vi "Configure_Voltage_Range.vi"(6 "Measurement Type":T2(ring), 8 "error in (no error)":errorcluster, 9 "Resolution in Digits":T1(ring), 10 "Range":dbl=1.2, 11 "NI-DCPower in":refnum<class "niDCPower.lvclass">) -> (0 "error out":errorcluster, 3 "NI-DCpower out":refnum<class "niDCPower.lvclass">)   [LabVIEW 2021, in "niDCPower.lvclass"]
uses:
  niDCPower.lvclass
  <instrlib>/niDCPower/nidcpower.llb/niDCPower Source Mode.ctl
  niDCPower.lvclass/niDCPower.ctl
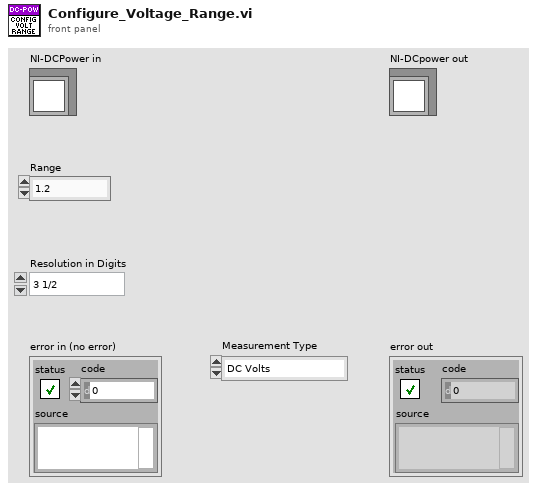
[diagram p1: front panel]
types:
  T1 = enum32{"3 1/2", "4 1/2", "5 1/2", "6 1/2", "7 1/2"}
  T2 = enum32{"DC Volts", "AC Volts", "DC Current", "AC Current", "2-wire Resistance", "4-wire Resistance", "Diode", "Frequency", "Period", "AC Volts DC Coupled", "Capacitance", "Inductance", "Temperature"}
  T3 = typedef "niDCPower Source Mode.ctl" = i32
  T4 = typedef "niDCPower Output Function.ctl" = i32
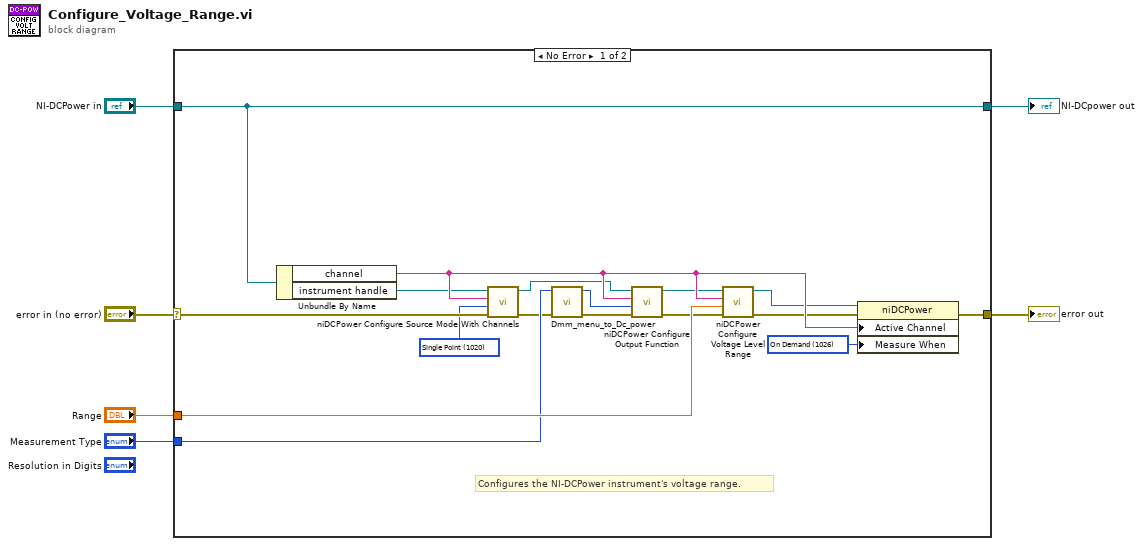
[diagram p0: block diagram]
diagram:
  n1 = case shown="No Error" "error in (no error)" {
    selector: "error in (no error)" -> [w23 w24]
    tunnel: [w22 w24] -> w5
    tunnel: "NI-DCPower in" -> [w19 w25]
    tunnel: [w19 w25] -> w3
    tunnel: "Range" -> [w21 _]
    tunnel: "Measurement Type" -> [w20 _]
    frame No Error {
      w12 = 1026 items=["Automatically after Source Complete"=1025, "On Demand"=1026, "On Measure Trigger"=1027] ("Measurement:Advanced:Measure When")
      w13 = T3 1020 items=["Single Point"=1020, "Sequence"=1021] ("source mode")
      # "Configures the NI-DCPower instrument's voltage range."
      n2 = Unbundle By Name(w19) -> ("channel"=w18:string, "instrument handle"=w17:refnum<k15>)
      n3 = call <instrlib>:"niDCPower Configure Source Mode With Channels.vi"("error in (no error)"=w23, "source mode"=w13, "channel name"=w18, "instrument handle"=w17) -> ("error out"=w10:errorcluster, "instrument handle out"=w16:refnum<k15>)  [unwired: 6 in]
      n4 = call "Dmm_menu_to_Dc_power.vi"("error in (no error)"=w10, "Measurement Type"=w20) -> ("error out"=w9:errorcluster, "output function"=w11:T4)  [unwired: 8 in]
      n5 = call <instrlib>:"niDCPower Configure Output Function.vi"("error in (no error)"=w9, "output function"=w11, "channel name"=w18, "instrument handle"=w16) -> ("error out"=w8:errorcluster, "instrument handle out"=w7:refnum<k15>)  [unwired: 6 out]
      n6 = call <instrlib>:"niDCPower Configure Voltage Level Range.vi"("error in (no error)"=w8, "voltage level range"=w21, "channel name"=w18, "instrument handle"=w7) -> ("error out"=w15:errorcluster, "instrument handle out"=w14:refnum<k15>)  [unwired: 6 out]
      n7 = property class="niDCPower"(reference=w14, error in=w15, "Active Channel"=w18, "Measure When"=w12) -> (error out=w22:errorcluster)  [unwired: 1 out]
    }
    frame Error {
    }
  }
  "error out" <- w5
  "NI-DCpower out" <- w3
